vi "DefenderCarla.vi"(7 "Field Size in":T1, 8 "Defensores":u32[](array[numeric]), 9 "Ball":dbl[](array[numeric]), 10 "total":i32) -> (2 "Posição dos Defensores":dbl[][](array[numeric]))   [LabVIEW 2016]
uses:
  Core/Field Size.ctl
panel:
  in  "Stretch":i32=60
  in  "Radius":i32=40
  in  "Array":dbl[][](array[numeric])=[[99999.0, 99999.0], [99999.0, 99999.0], [99999.0, 99999.0], [99999.0, 99999.0], [99999.0, 99999.0]]
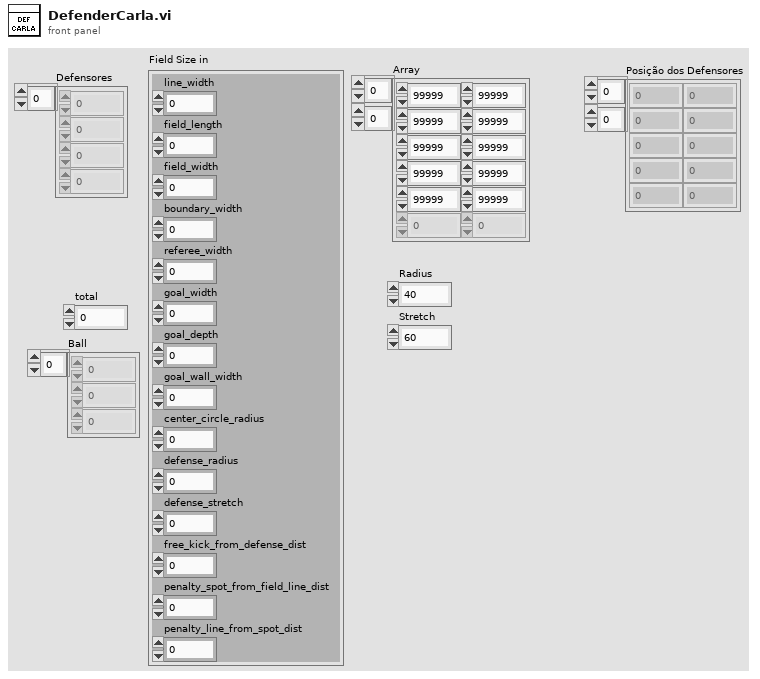
[diagram p1: front panel]
types:
  T1 = typedef "Field Size.ctl" = cluster{"line_width":u32, "field_length":u32, "field_width":u32, "boundary_width":u32, "referee_width":u32, "goal_width":u32, "goal_depth":u32, "goal_wall_width":u32, "center_circle_radius":u32, "defense_radius":u32, "defense_stretch":u32, "free_kick_from_defense_dist":u32, "penalty_spot_from_field_line_dist":u32, "penalty_line_from_spot_dist":u32}
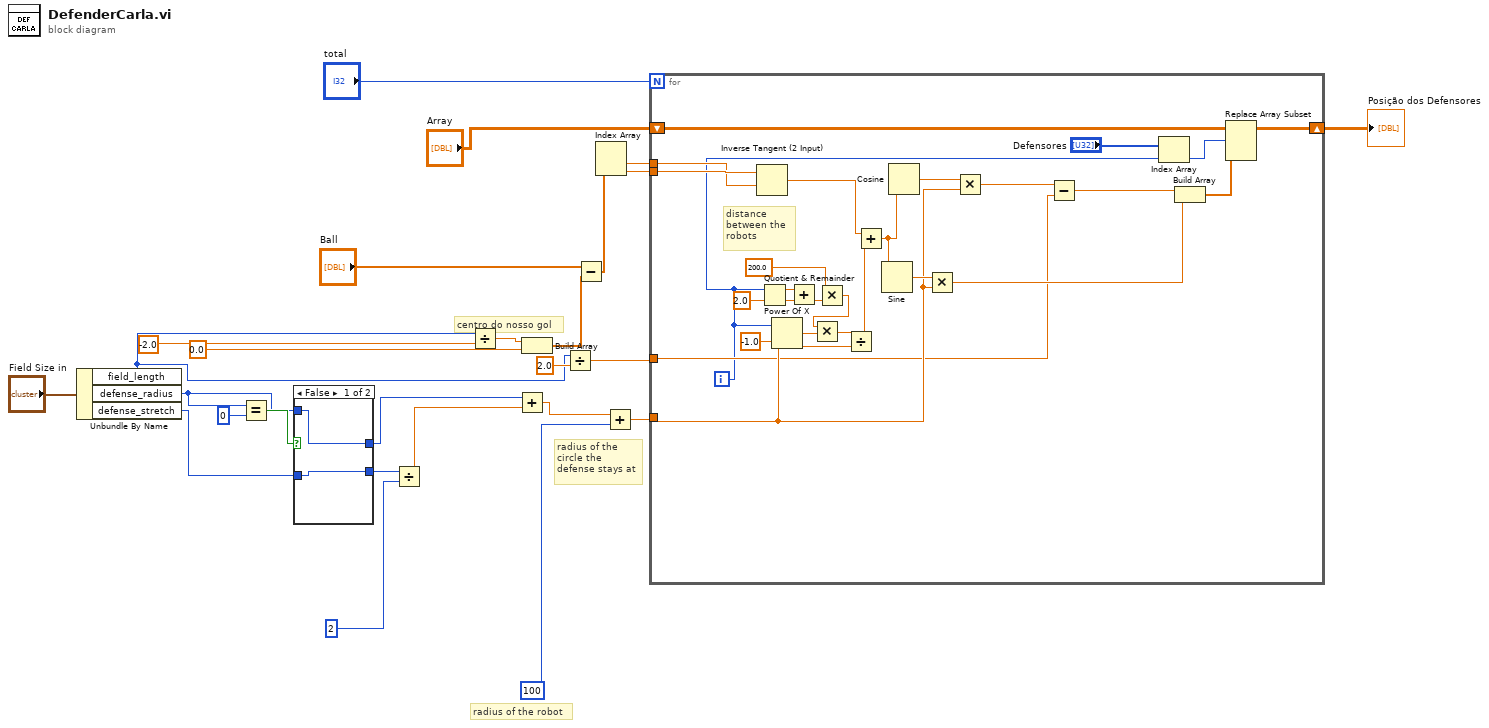
[diagram p0: block diagram]
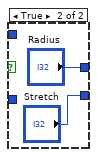
[diagram p2: hidden frame]
diagram:
  # "radius of the circle the defense stays at"
  # "centro do nosso gol"
  # "radius of the robot"
  n1 = Unbundle By Name("Field Size in") -> ("field_length"=w10:u32, "defense_radius"=w3:u32, "defense_stretch"=w2:u32)
  n2 = Equal?(x=w3, y=u32 0) -> (x = y?=w5:bool)
  n3 = case shown="False" w5 {
    tunnel: [w28 "Radius"] -> w4
    tunnel: w3 -> [w28 _]
    tunnel: w2 -> [w27 _]
    tunnel: [w27 "Stretch"] -> w1
    frame False {
    }
    frame True {
    }
  }
  n4 = Divide(x=w1, y=u32 2) -> (x/y=w13:dbl)
  n5 = Divide(x=w10, y=-2.0) -> (x/y=w22:dbl)
  n6 = Add(x=w4, y=w13) -> (x+y=w25:dbl)
  n7 = Build Array(w22, 0.0 ("element")) -> (w18:dbl[])
  n8 = Divide(x=w10, y=2.0) -> (x/y=w9:dbl)
  n9 = Subtract(x="Ball", y=w18) -> (x-y=w17:dbl[])
  n10 = Index Array(array=w17) -> (element #1=w15:dbl, element #2=w16:dbl)  [unwired: 2 in]
  n11 = Add(x=w25, y=u32 100) -> (x+y=w14:dbl)
  n12 = for {
    N: "total" -> [_]
    tunnel: w16 -> [w57]
    tunnel: w15 -> [w56]
    tunnel: w14 -> [w46]
    shift-right: [w34] -> w8
    shift-left: "Array" -> [w33]
    tunnel: w9 -> [w43]
    i -> [w32]
    # "distance between the robots"
    n13 = Inverse Tangent (2 Input)(1:w56, 2:w57) -> (0:w52:dbl)
    n14 = Quotient & Remainder(x=w32, y=2.0) -> (x-y*floor(x/y)=w39:dbl, floor(x/y)=w38:dbl)
    n15 = Power Of X(1:-1.0, 2:w32) -> (0:w54:dbl)
    n16 = Add(x=w39, y=w38) -> (x+y=w37:dbl)
    n17 = Multiply(x=200.0, y=w37) -> (x*y=w41:dbl)
    n18 = Multiply(x=w41, y=w54) -> (x*y=w53:dbl)
    n19 = Divide(x=w53, y=w46) -> (x/y=w51:dbl)
    n20 = Add(x=w52, y=w51) -> (x+y=w50:dbl)
    n21 = Sine(x=w50) -> (sin(x)=w48:dbl)
    n22 = Cosine(x=w50) -> (cos(x)=w49:dbl)
    n23 = Multiply(x=w48, y=w46) -> (x*y=w44:dbl)
    n24 = Multiply(x=w49, y=w46) -> (x*y=w47:dbl)
    n25 = Subtract(x=w47, y=w43) -> (x-y=w45:dbl)
    n26 = Index Array(array="Defensores", index=w32) -> (element=w31:u32)
    n27 = Build Array(w45, w44) -> (w35:dbl[])
    n28 = Replace Array Subset(array=w33, new element=w35, index (row)=w31) -> (w34:dbl[][])  [unwired: 1 in]
  }
  "Posição dos Defensores" <- w8
